vi "Read States.vi"(8 "error in (no error)":errorcluster, 11 "PenaltyTactic in":refnum<class "PenaltyTactic.lvclass">) -> (0 "error out":errorcluster, 2 "States":T1(ring), 3 "PenaltyTactic out":refnum<class "PenaltyTactic.lvclass">)   [LabVIEW 2021, in "PenaltyTactic.lvclass"]
uses:
  PenaltyTactic.lvclass
  PenaltyTactic.lvclass/PenaltyTactic.ctl
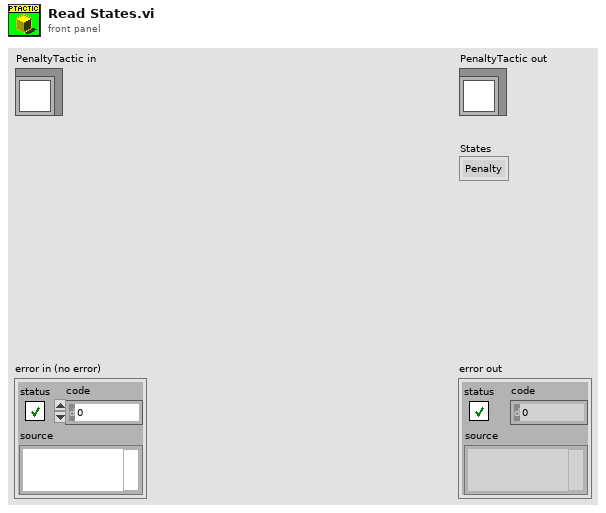
[diagram p1: front panel]
types:
  T1 = enum16{"Penalty", "Kick", "Pos3", "Pos2", "Pos1", "Exit"}
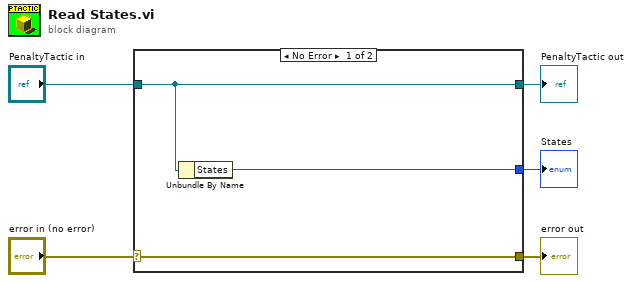
[diagram p0: block diagram]
diagram:
  n1 = case shown="No Error" "error in (no error)" {
    selector: "error in (no error)" -> [w8 w9]
    tunnel: [w8 w9] -> w4
    tunnel: [w7 w10] -> w2
    tunnel: "PenaltyTactic in" -> [w7 w10]
    tunnel: [w6 _] -> w1
    frame No Error {
      n2 = Unbundle By Name(w7) -> ("States"=w6:T1)
    }
    frame Error {
    }
  }
  "error out" <- w4
  "PenaltyTactic out" <- w2
  "States" <- w1
